vi "Counter.vi"() -> ()   [LabVIEW 2012]
uses:
  <vilib>/DAQmx/read.llb/DAQmx Read (Counter U32 1Chan 1Samp).vi
  <vilib>/DAQmx/create/channels.llb/DAQmx Create Channel (CI-Count Edges).vi
  <vilib>/DAQmx/miscellaneous.llb/DAQmx Fill In Error Info.vi
panel:
  out "Det1":u32
  out "Det2":u32
  out "Det3":u32
  out "PSU":u32
  out "error out":errorcluster
  in  "PSU":tag="Dev4/ctr1"
  in  "Det3":tag="Dev4/ctr0"
  in  "Det2":tag="Dev5/ctr1"
  in  "Det1":tag="Dev5/ctr0"
  in  "stop":bool
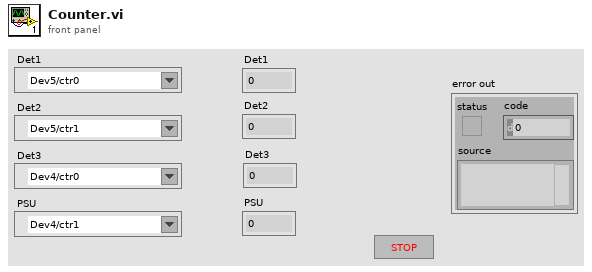
[diagram p1: front panel]
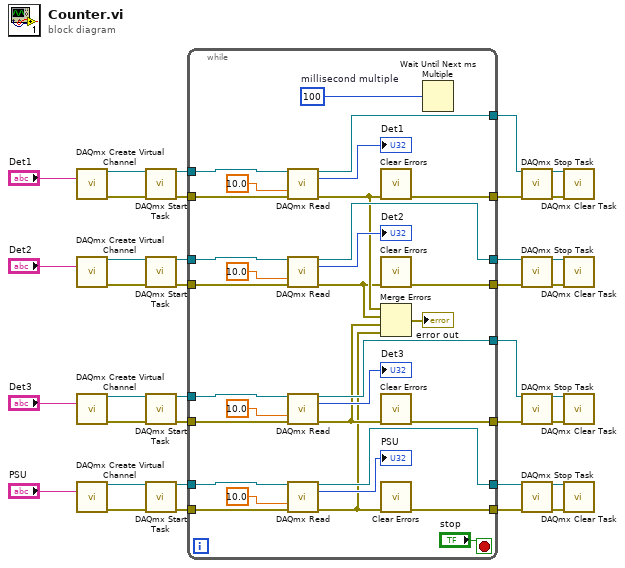
[diagram p0: block diagram]
diagram:
  n1 = call-poly <vilib>:"DAQmx Create Virtual Channel.vi"("counter"="Det1") -> ("task out"=w8:refnum<k21>, "error out"=w1:errorcluster)  [unwired: 13 in]
  n2 = call-poly <vilib>:"DAQmx Create Virtual Channel.vi"("counter"="Det2") -> ("task out"=w7:refnum<k21>, "error out"=w2:errorcluster)  [unwired: 13 in]
  n3 = call-poly <vilib>:"DAQmx Create Virtual Channel.vi"("counter"="Det3") -> ("task out"=w6:refnum<k21>, "error out"=w5:errorcluster)  [unwired: 13 in]
  n4 = call-poly <vilib>:"DAQmx Create Virtual Channel.vi"("counter"="PSU") -> ("task out"=w4:refnum<k21>, "error out"=w3:errorcluster)  [unwired: 13 in]
  n5 = call <vilib>:"DAQmx Start Task.vi"("task/channels in"=w8, "error in"=w1) -> ("task out"=w32:refnum<k21>, "error out"=w25:errorcluster)  [unwired: 12 in]
  n6 = call <vilib>:"DAQmx Start Task.vi"("task/channels in"=w7, "error in"=w2) -> ("task out"=w31:refnum<k21>, "error out"=w26:errorcluster)  [unwired: 12 in]
  n7 = call <vilib>:"DAQmx Start Task.vi"("task/channels in"=w6, "error in"=w5) -> ("task out"=w30:refnum<k21>, "error out"=w27:errorcluster)  [unwired: 12 in]
  n8 = call <vilib>:"DAQmx Start Task.vi"("task/channels in"=w4, "error in"=w3) -> ("task out"=w29:refnum<k21>, "error out"=w28:errorcluster)  [unwired: 12 in]
  n9 = while {
    tunnel: w32 -> [w67]
    tunnel: w31 -> [w60]
    tunnel: w30 -> [w58]
    tunnel: w29 -> [w56]
    tunnel: w28 -> [w55]
    tunnel: w27 -> [w57]
    tunnel: w26 -> [w59]
    tunnel: w25 -> [w66]
    tunnel: [w65] -> w24
    tunnel: [w47] -> w23
    tunnel: [w50] -> w22
    tunnel: [w46] -> w21
    tunnel: [w45] -> w19
    tunnel: [w49] -> w20
    tunnel: [w48] -> w18
    tunnel: [w44] -> w17
    stop <- "stop" stop-if-true
    w43 = u32 100  # millisecond multiple
    n10 = call-poly <vilib>:"DAQmx Read.vi"("task/channels in"=w67, "timeout"=10.0, "error in"=w66) -> ("task out"=w65:refnum<k21>, "data"=→"Det1":u32, "error out"=w41:errorcluster)  [unwired: 10 in]
    n11 = call-poly <vilib>:"DAQmx Read.vi"("task/channels in"=w60, "timeout"=10.0, "error in"=w59) -> ("task out"=w50:refnum<k21>, "data"=→"Det2":u32, "error out"=w40:errorcluster)  [unwired: 10 in]
    n12 = call-poly <vilib>:"DAQmx Read.vi"("task/channels in"=w58, "timeout"=10.0, "error in"=w57) -> ("task out"=w49:refnum<k21>, "data"=→"Det3":u32, "error out"=w39:errorcluster)  [unwired: 10 in]
    n13 = call-poly <vilib>:"DAQmx Read.vi"("task/channels in"=w56, "timeout"=10.0, "error in"=w55) -> ("task out"=w48:refnum<k21>, "data"=→"PSU":u32, "error out"=w38:errorcluster)  [unwired: 10 in]
    n14 = call <vilib>:"Clear Errors.vi"("error in (no error)"=w41) -> ("error out"=w47:errorcluster)  [unwired: 6 in]
    n15 = call <vilib>:"Clear Errors.vi"("error in (no error)"=w40) -> ("error out"=w46:errorcluster)  [unwired: 6 in]
    n16 = Merge Errors(w41, w40, w39, w38) -> (→"error out":errorcluster)
    n17 = call <vilib>:"Clear Errors.vi"("error in (no error)"=w39) -> ("error out"=w45:errorcluster)  [unwired: 6 in]
    n18 = call <vilib>:"Clear Errors.vi"("error in (no error)"=w38) -> ("error out"=w44:errorcluster)  [unwired: 6 in]
    n19 = Wait Until Next ms Multiple(millisecond multiple=w43) -> ()  [unwired: 1 out]
  }
  n20 = call <vilib>:"DAQmx Stop Task.vi"("task/channels in"=w24, "error in"=w23) -> ("task out"=w16:refnum<k21>, "error out"=w15:errorcluster)  [unwired: 12 in]
  n21 = call <vilib>:"DAQmx Stop Task.vi"("task/channels in"=w22, "error in"=w21) -> ("task out"=w14:refnum<k21>, "error out"=w13:errorcluster)  [unwired: 12 in]
  n22 = call <vilib>:"DAQmx Stop Task.vi"("task/channels in"=w20, "error in"=w19) -> ("task out"=w12:refnum<k21>, "error out"=w11:errorcluster)  [unwired: 12 in]
  n23 = call <vilib>:"DAQmx Stop Task.vi"("task/channels in"=w18, "error in"=w17) -> ("task out"=w10:refnum<k21>, "error out"=w9:errorcluster)  [unwired: 12 in]
  n24 = call <vilib>:"DAQmx Clear Task.vi"("task in"=w16, "error in"=w15) -> ()  [unwired: 13 in, 1 out]
  n25 = call <vilib>:"DAQmx Clear Task.vi"("task in"=w14, "error in"=w13) -> ()  [unwired: 13 in, 1 out]
  n26 = call <vilib>:"DAQmx Clear Task.vi"("task in"=w12, "error in"=w11) -> ()  [unwired: 13 in, 1 out]
  n27 = call <vilib>:"DAQmx Clear Task.vi"("task in"=w10, "error in"=w9) -> ()  [unwired: 13 in, 1 out]
